vi "WS Action and Status.vi"() -> ()   [LabVIEW 2020]
uses:
  WS Admin/Scheme.ctl
  WS Admin/WS Action.ctl
  WS Admin/WS Status.ctl
  WS Admin/WS Admin.lvlib
panel:
  out "Status After":T1
  out "Status Before":T1
  out "error out":errorcluster
  in  "Port":u16
  in  "Host":string
  in  "Action":T2
  in  "WS Name":string
  in  "Scheme":T3
  # "Fill these out and then run the VI"
  # "1."
  # "2."
  # "3."
  # "1. Enter the server connection info which will be found either in the Application Web Server deployment settings for the web service or in the NI Web Server configuration application.\n\n2. The name for the WS. This should match the name displayed in the web service administration page which may be slightly different as LabVIEW removes/replaces special characters in names.\n\n3. Select which action to perform on the Web Service."
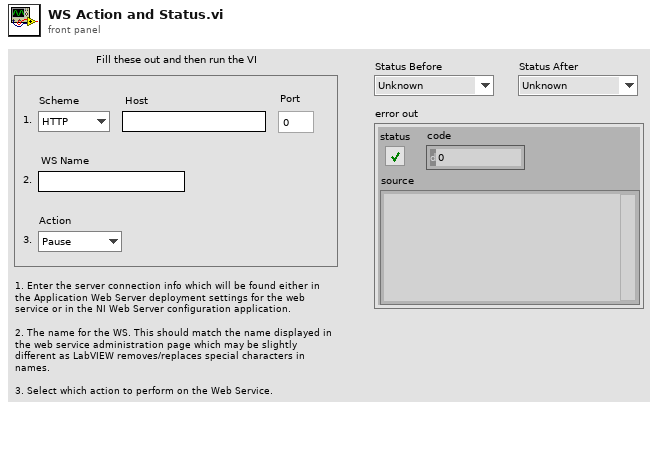
[diagram p1: front panel]
types:
  T1 = typedef "WS Admin.lvlib/WS Status.ctl" = enum16{"Unknown", "Paused", "Running"}
  T2 = typedef "WS Admin.lvlib/WS Action.ctl" = enum16{"Pause", "Resume", "Restart", "Unpublish"}
  T3 = typedef "WS Admin.lvlib/Scheme.ctl" = enum16{"HTTP", "HTTPS"}
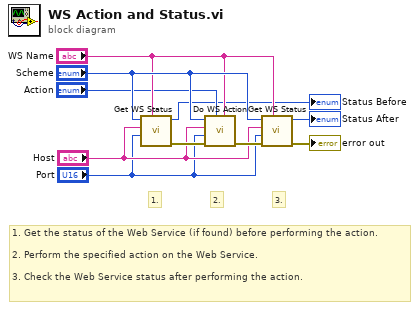
[diagram p0: block diagram]
diagram:
  # "1. Get the status of the Web Service (if found) before performing the action.\n\n2. Perform the specified action on the Web Service.\n\n3. Check the Web Service status after performing the action."
  # "3."
  # "2."
  # "1."
  n1 = call "Get WS Status.vi"("WS Name"="WS Name", "Port"="Port", "Host"="Host", "Scheme (HTTP)"="Scheme") -> ("error out"=w10:errorcluster, "Status"=→"Status Before":T1)  [unwired: 6 in]
  n2 = call "Do WS Action.vi"("WS Name"="WS Name", "Action"="Action", "error in (no error)"=w10, "Port"="Port", "Host"="Host", "Scheme (HTTP)"="Scheme") -> ("error out"=w9:errorcluster)  [unwired: 5 in]
  n3 = call "Get WS Status.vi"("WS Name"="WS Name", "error in (no error)"=w9, "Port"="Port", "Host"="Host", "Scheme (HTTP)"="Scheme") -> ("error out"=→"error out":errorcluster, "Status"=→"Status After":T1)  [unwired: 5 in]
